vi "Validate API method.vi"(8 "error in (no error)":errorcluster, 10 "Command in":variant, 11 "Instrument in":refnum<class "Instrument.lvclass">) -> (0 "error out":errorcluster, 2 "command out":string, 3 "Instrument out":refnum<class "Instrument.lvclass">)   [LabVIEW 2019, in "Instrument.lvclass"]
uses:
  Instrument.lvclass
  fc7ddfc3-4691-44af-af0a-414f479c60a8.vi
  <vilib>/Utility/Data Type/Get Numeric Information.vi
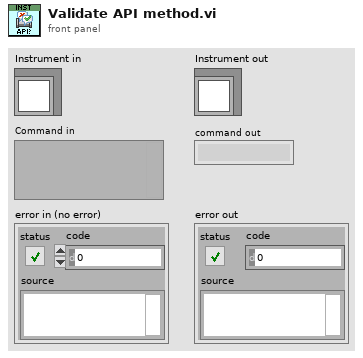
[diagram p1: front panel]
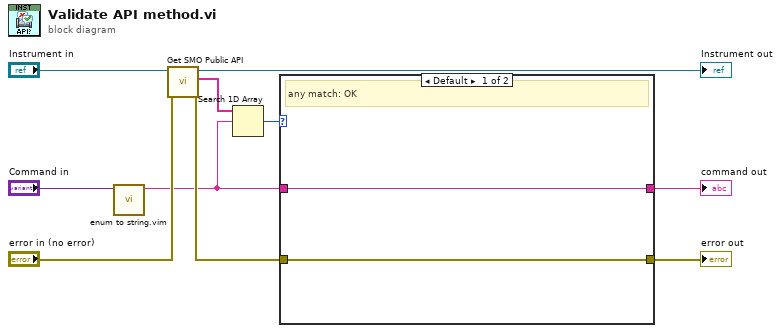
[diagram p0: block diagram]
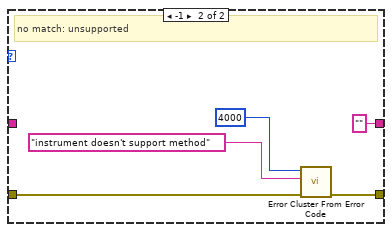
[diagram p2: hidden frame]
diagram:
  n1 = call "enum to string.vim"("enum in"="Command in") -> ("string out"=w1:string)  [unwired: 9 in, 1 out]
  n2 = call-dynamic "Get SMO Public API.vi"("error in (no error)"="error in (no error)", "Instrument in"="Instrument in") -> ("error out"=w5:errorcluster, "Commands"=w7:string[], "Instrument out"=→"Instrument out":refnum<class "Instrument.lvclass">)  [unwired: 7 in]
  n3 = Search 1D Array(1D array=w7, element=w1) -> (index of element=w9:i32)  [unwired: 1 in]
  n4 = case shown="Default" w9 {
    tunnel: [w12 w15] -> w10
    tunnel: w5 -> [w12 w14]
    tunnel: [w11 "" ("command in")] -> w8
    tunnel: w1 -> [w11 _]
    frame Default {
      # "any match: OK"
    }
    frame -1 {
      # "no match: unsupported"
      n5 = call <vilib>:"Error Cluster From Error Code.vi"("error in (no error)"=w14, "error message (\"\")"="instrument doesn't support method" ("error message (\"\")"), "error code (0)"=4000) -> ("error out"=w15:errorcluster)  [unwired: 6 in]
    }
  }
  "error out" <- w10
  "command out" <- w8
